vi "FilterDynamixelTorque.vi"(8 "Queue timeout (ms)":i32=200, 10 "DynamixelTorque Queue":refnum<queue>, 11 "NotifierReff":T1) -> ()   [LabVIEW 2013]
doc: "Performs and filtering that we want (default is no filtering) and writes the data to the notifier. If no data is in the queue this VI times out after 'Queue timeout (ms)' has passed and nothing is written to the notifier. When only one Dynamixel times, then '-1' is written to the timed out Dynamixel and the other torque is written to the notifier.\n\nEric Schneider, March 2014"
uses:
  Data/TypeDefs/Notifiers.ctl
  Data/TypeDefs/UTM Location.ctl
  Data/TypeDefs/Sail Set Suggestions.ctl
  Data/TypeDefs/Rudder Set Suggestions.ctl
  Data/TypeDefs/OverrideInformation.ctl
  Data/TypeDefs/OverrideMode.ctl
  Data/TypeDefs/MotorSetup.ctl
  Data/TypeDefs/DynamixelSetupInfo.ctl
  Data/TypeDefs/AirmarStatus.ctl
  Data/TypeDefs/HardwareOnline.ctl
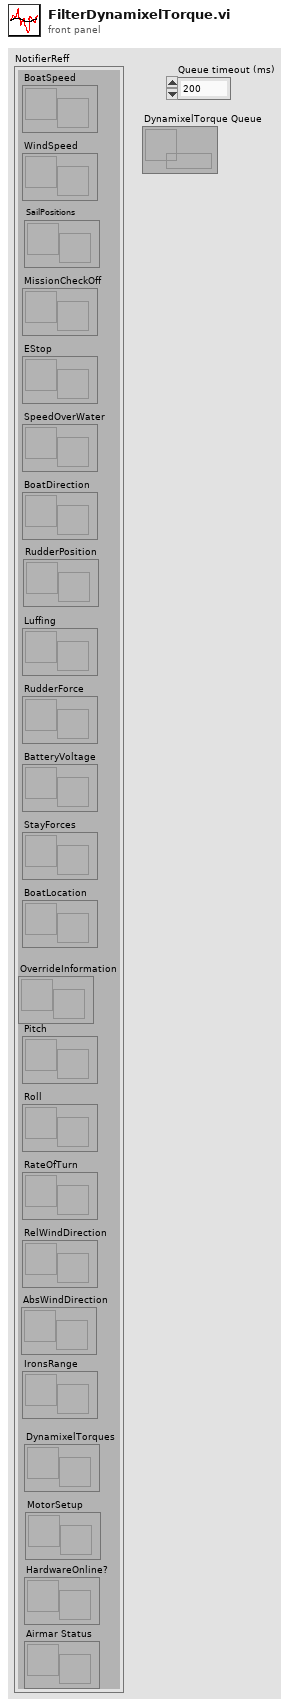
[diagram p1: front panel]
types:
  T1 = typedef "Notifiers.ctl" = cluster{"BoatSpeed":refnum<notifier>, "WindSpeed":refnum<notifier>, "MissionCheckOff":refnum<notifier>, "EStop":refnum<notifier>, "SpeedOverWater":refnum<notifier>, "BoatDirection":refnum<notifier>, "Luffing":refnum<notifier>, "RudderForce":refnum<notifier>, "BatteryVoltage":refnum<notifier>, "StayForces":refnum<notifier>, "BoatLocation":refnum<notifier>, "Pitch":refnum<notifier>, "Roll":refnum<notifier>, "RateOfTurn":refnum<notifier>, "RelWindDirection":refnum<notifier>, "SailPositions":refnum<notifier>, "RudderPosition":refnum<notifier>, "IronsRange":refnum<notifier>, "AbsWindDirection":refnum<notifier>, "OverrideInformation":refnum<notifier>, "DynamixelTorques":refnum<notifier>, "MotorSetup":refnum<notifier>, "Airmar Status":refnum<notifier>, "HardwareOnline?":refnum<notifier>}
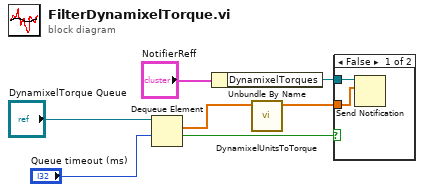
[diagram p0: block diagram]
diagram:
  n1 = Dequeue Element(queue="DynamixelTorque Queue", timeout in ms (-1)="Queue timeout (ms)") -> (element=w3:dbl[], timed out?=w1:bool)  [unwired: 1 in, 2 out]
  n2 = Unbundle By Name("NotifierReff") -> ("DynamixelTorques"=w6:refnum<notifier>)
  n3 = call "DynamixelUnitsToTorque.vi"("Dynamixel values"=w3) -> ("Torque on Dynamixel (N*m)"=w2:dbl[])  [unwired: 10 in]
  n4 = case shown="False" w1 {
    tunnel: w6 -> [w9 _]
    tunnel: w2 -> [w8 _]
    frame False {
      n5 = Send Notification(notification=w8, notifier=w9) -> ()  [unwired: 1 in, 2 out]
    }
    frame True {
    }
  }
